vi "Motor_Begin.vi"   [LabVIEW 2014]
uses:
  <vilib>/Rock Robotics/WPI/SafetyOutput/WPI_SafetyOutputConfigMenu.ctl
  <vilib>/Rock Robotics/WPI/CAN/TalonSRX/WPI_CANTalonSRX_APIControlMode.ctl
  <vilib>/Rock Robotics/WPI/MotorControl/WPI_MotorControlOpenCANTalonSRX.vi
  <vilib>/Rock Robotics/WPI/RobotDrive/WPI_RobotDriveOpen4MotorWithCANTalonSRX.vi
types:
  T1 = typedef "WPI_CANTalonSRX_APIControlMode.ctl" = enum8{"Percent VBus", "Speed", "Position", "Slave", "Unchanged / Invalid"}
  T2 = typedef "WPI_SafetyOutputConfigMenu.ctl" = enum16{"Enable", "Disable"}
  T3 = typedef "WPI_MotorControlDeviceRef.ctl" = cluster{"DeviceStatus":errorcluster, "Type":T4, "PWM":cluster{"Controller":T5, "PWM Channel":T6, "DeadBand":T7}, "CAN":cluster{"Device Number":u8, "Control Mode":T8, "Semaphore":T9, "Max Vout":dbl, "TalonSRX Control Mode":T1}, "Invert":bool, "TransformRef":T10, "InvTransformRef":T10}
  T4 = typedef "WPI_MotorControlType.ctl" = enum16{"PWM", "CAN", "CANTalonSRX"}
  T5 = typedef "FPGA_TypedefDigitalModule.ctl" = enum16{"Controller 1"}
  T6 = typedef "FPGA_DIOPWMChannel.ctl" = enum8{"PWM 0", "PWM 1", "PWM 2", "PWM 3", "PWM 4", "PWM 5", "PWM 6", "PWM 7", "PWM 8", "PWM 9", "PWM MXP 0", "PWM MXP 1", "PWM MXP 2", "PWM MXP 3", "PWM MXP 4", "PWM MXP 5", "PWM MXP 6", "PWM MXP 7", "PWM MXP 8", "PWM MXP 9", "Invalid"}
  T7 = typedef "WPI_PWMDeadband.ctl" = cluster{"Name":string, "maxPositivePwm":i32, "minPositivePwm":i32, "centerPwm":i32, "maxNegativePwm":i32, "minNegativePwm":i32, "angularRange":u16}
  T8 = typedef "WPI_CANJaguar_ControlMode.ctl" = enum8{"Percent VBus", "Current", "Speed", "Position", "Voltage"}
  T9 = typedef "Semaphore RefNum" = refnum<k1>
  T10 = typedef "WPI_PWMTransform_ConPane.ctl" = refnum<vi>
  T11 = typedef "WPI_RobotDriveDevRef.ctl" = cluster{"DevStatus":errorcluster, "Motors[]":T3[], "Square Inputs":bool, "Max Output":dbl}
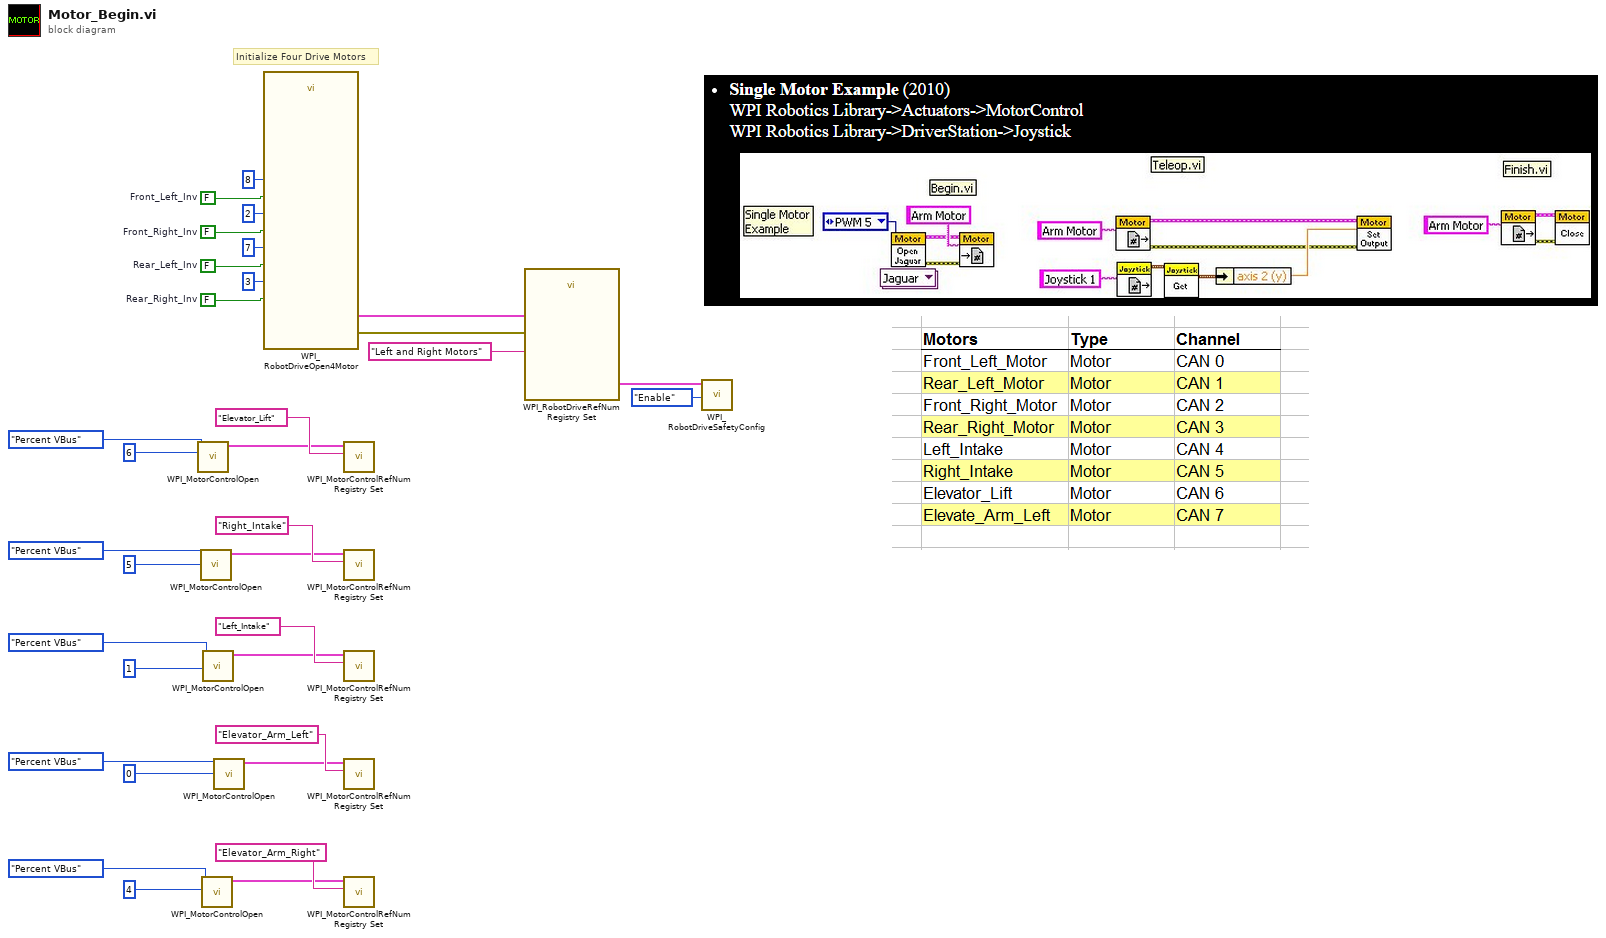
[diagram p0: block diagram]
diagram:
  w23 = FALSE  # Rear_Right_Inv
  w22 = FALSE  # Rear_Left_Inv
  w21 = FALSE  # Front_Right_Inv
  w20 = FALSE  # Front_Left_Inv
  # "Initialize Four Drive Motors"
  n1 = call-poly <vilib>:"WPI_MotorControlOpen.vi"("Device Number"=u8 6, "Control Mode"=WPI_CANTalonSRX_APIControlMode."Percent VBus") -> ("MotorControlDeviceRef"=w28:T3)  [unwired: 8 in, 1 out]
  n2 = call-poly <vilib>:"WPI_MotorControlOpen.vi"("Device Number"=u8 5, "Control Mode"=WPI_CANTalonSRX_APIControlMode."Percent VBus") -> ("MotorControlDeviceRef"=w26:T3)  [unwired: 8 in, 1 out]
  n3 = call-poly <vilib>:"WPI_MotorControlOpen.vi"("Device Number"=u8 4, "Control Mode"=WPI_CANTalonSRX_APIControlMode."Percent VBus") -> ("MotorControlDeviceRef"=w32:T3)  [unwired: 8 in, 1 out]
  n4 = call-poly <vilib>:"WPI_MotorControlOpen.vi"("Device Number"=u8 1, "Control Mode"=WPI_CANTalonSRX_APIControlMode."Percent VBus") -> ("MotorControlDeviceRef"=w24:T3)  [unwired: 8 in, 1 out]
  n5 = call-poly <vilib>:"WPI_MotorControlOpen.vi"("Device Number"=u8 0, "Control Mode"=WPI_CANTalonSRX_APIControlMode."Percent VBus") -> ("MotorControlDeviceRef"=w30:T3)  [unwired: 8 in, 1 out]
  n6 = call-poly <vilib>:"WPI_RobotDriveOpen4Motor.vi"("Rear Left Motor"=u8 7 ("Rear Right Motor"), "Rear Left Motor Inverted"=w22, "Rear Right Motor Inverted"=w23, "Rear Right Motor"=u8 3 ("Front Left Motor"), "Front Left Motor"=u8 8 ("Front Right Motor"), "Front Right Motor"=u8 2 ("Rear Left Motor"), "Front Left Motor Inverted"=w20, "Front Right Motor Inverted"=w21) -> ("RobotDriveDevRef"=w18:T11, "error out"=w17:errorcluster)  [unwired: 6 in]
  n7 = call <vilib>:"WPI_MotorControlRefNum Registry Set.vi"("refnum name"="Elevator_Lift", "MotorControlDevRef"=w28) -> ()  [unwired: 8 in, 2 out]
  n8 = call <vilib>:"WPI_MotorControlRefNum Registry Set.vi"("refnum name"="Right_Intake", "MotorControlDevRef"=w26) -> ()  [unwired: 8 in, 2 out]
  n9 = call <vilib>:"WPI_MotorControlRefNum Registry Set.vi"("refnum name"="Left_Intake", "MotorControlDevRef"=w24) -> ()  [unwired: 8 in, 2 out]
  n10 = call <vilib>:"WPI_MotorControlRefNum Registry Set.vi"("refnum name"="Elevator_Arm_Left", "MotorControlDevRef"=w30) -> ()  [unwired: 8 in, 2 out]
  n11 = call <vilib>:"WPI_MotorControlRefNum Registry Set.vi"("refnum name"="Elevator_Arm_Right", "MotorControlDevRef"=w32) -> ()  [unwired: 8 in, 2 out]
  n12 = call <vilib>:"WPI_RobotDriveRefNum Registry Set.vi"("error in (no error)"=w17, "refnum name"="Left and Right Motors", "RobotDriveDevRef"=w18) -> ("RobotDriveDevRef"=w15:T11)  [unwired: 8 out]
  n13 = call <vilib>:"WPI_RobotDriveSafetyConfig.vi"("mode"=WPI_SafetyOutputConfigMenu."Enable", "RobotDriveDevRef"=w15) -> ()  [unwired: 8 in, 2 out]
